vi "fgv_sessions.vi"(7 "Operation":T2(ring), 8 "error in":errorcluster, 10 "Session User Data in (None)":T1={"Instr type"="", "Instr type for err. msg."="", "Installed Options"=[], "OPC Timeout"=5000, "Query Instrument Status"=TRUE, "Check Range"=TRUE, "Check Options"=TRUE, "Add LF to Write"=TRUE, "Simulate"=FALSE, "Logging"=FALSE, "Logging params"=variant, "Interface Type"=enum."GPIB_VXI", "Fast Sweep"=0, "AdditionalFlags"=5000, "WaitBeforeWrite"=0, "WaitBeforeRead"=0, "BinDataChunkSize"=10000000} {"BinDataChunkSize" format="%.0p"; "AdditionalFlags" format="%08b"; "Fast Sweep" items=["Normal", "Fast"]}, 11 "VISA resource name":refnum<visa-resource-name>) -> (0 "error out":errorcluster, 2 "Session User Data out":T1={"Instr type"="", "Instr type for err. msg."="", "Installed Options"=[], "OPC Timeout"=5000, "Query Instrument Status"=TRUE, "Check Range"=TRUE, "Check Options"=TRUE, "Add LF to Write"=TRUE, "Simulate"=FALSE, "Logging"=FALSE, "Logging params"=variant, "Interface Type"=enum."GPIB_VXI", "Fast Sweep"=0, "AdditionalFlags"=5000, "WaitBeforeWrite"=0, "WaitBeforeRead"=0, "BinDataChunkSize"=10000000} {"BinDataChunkSize" format="%.0p"; "AdditionalFlags" format="%08b"; "Fast Sweep" items=["Normal", "Fast"]}, 3 "VISA resource name out":refnum<visa-resource-name> caption="VISA resource name")   [LabVIEW 2014, in "rszvl_rsidr_core.lvlib"]
uses:
  rszvl_rsidr_core.lvlib
  type_Session_Data.ctl
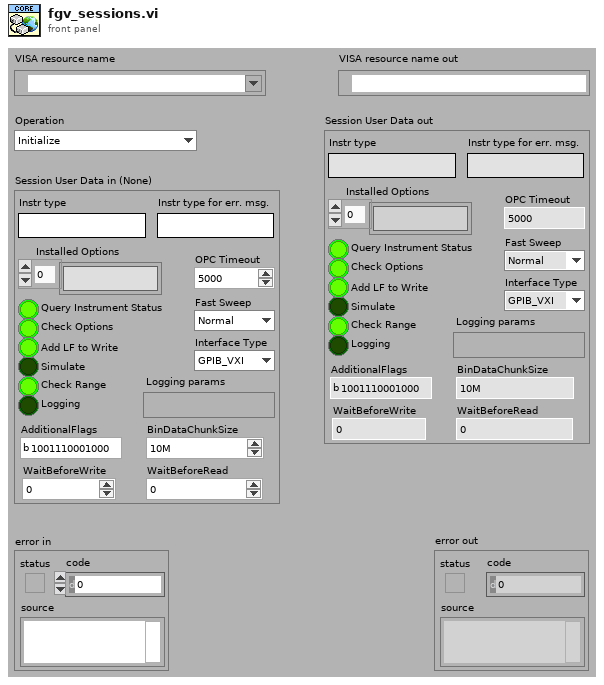
[diagram p1: front panel]
types:
  T1 = typedef "rszvl_rsidr_core.lvlib/type_Session_Data.ctl" = cluster{"Instr type":string, "Instr type for err. msg.":string, "Installed Options":string[], "OPC Timeout":i32, "Query Instrument Status":bool, "Check Range":bool, "Check Options":bool, "Add LF to Write":bool, "Simulate":bool, "Logging":bool, "Logging params":variant, "Interface Type":enum16{"Unknown", "GPIB", "VXI", "GPIB_VXI", "ASRL", "PXI", "TCPIP", "USB", "SOCKET"}, "Fast Sweep":i32, "AdditionalFlags":i32, "WaitBeforeWrite":i32, "WaitBeforeRead":i32, "BinDataChunkSize":i64}
  T2 = enum16{"Initialize", "GetData", "SetData", "Clear"}
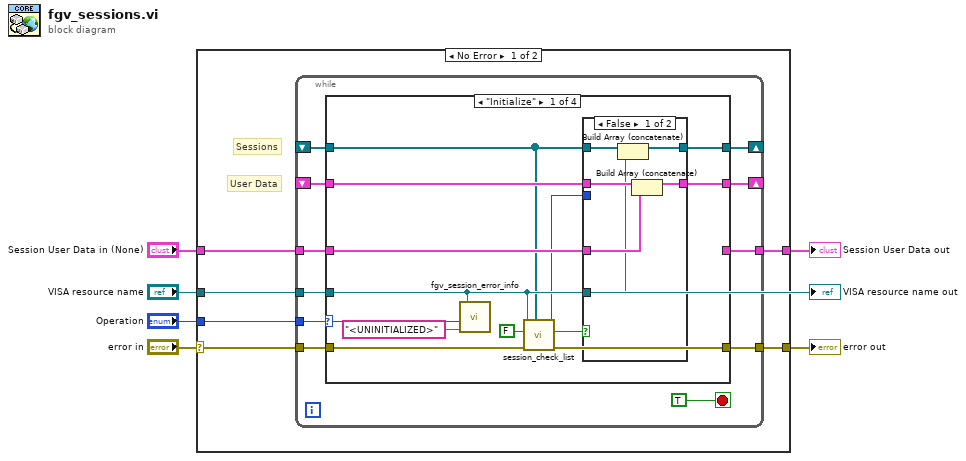
[diagram p0: block diagram]
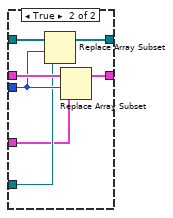
[diagram p2: hidden frame]
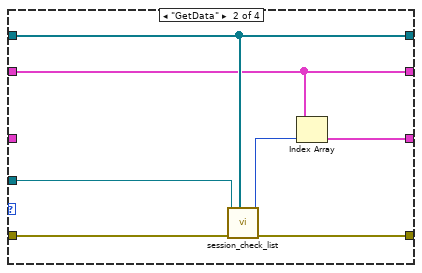
[diagram p3: hidden frame]
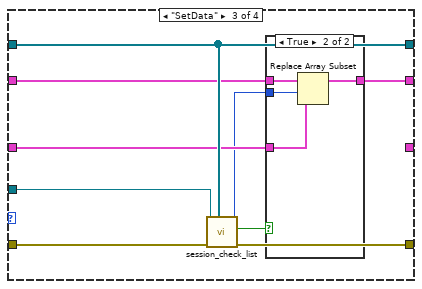
[diagram p4: hidden frame]
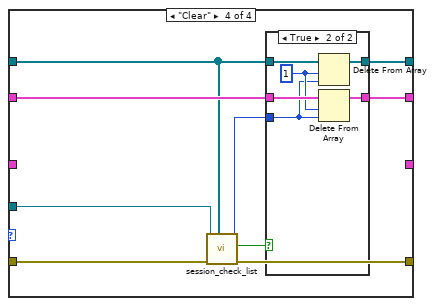
[diagram p6: hidden frame]
diagram:
  n1 = case shown="No Error" "error in" {
    selector: "error in" -> [w11 w88]
    tunnel: "Operation" -> [w8 _]
    tunnel: "Session User Data in (None)" -> [w9 _]
    tunnel: "VISA resource name" -> [w7 _]
    tunnel: [w12 _] -> w5
    tunnel: [w10 w88] -> w1
    frame No Error {
      # "User Data"
      # "Sessions"
      n2 = while {
        tunnel: [w13] -> w12
        tunnel: w11 -> [w16]
        tunnel: [w23] -> w10
        tunnel: w9 -> [w22]
        tunnel: w8 -> [w21]
        tunnel: w7 -> [w20]
        shift-right: [w18] -> _
        shift-left: _ -> [w19]
        shift-right: [w14] -> _
        shift-left: _ -> [w15]
        stop <- TRUE stop-if-true
        n3 = case "Operation case" shown="\"Initialize\"" w21 {
          selector: w21 -> [w25 _ _ _]
          tunnel: w20 -> [w26 w54 w64 w78]
          tunnel: w16 -> [w36 w56 w65 w79]
          tunnel: [w35 w55 w59 w77] -> w23
          tunnel: w19 -> [w30 w53 w63 w72]
          tunnel: w22 -> [w31 _ w61 _]
          tunnel: [w29 w53 w63 w71] -> w18
          tunnel: w15 -> [w32 w51 w62 w76]
          tunnel: [w28 w51 w60 w73] -> w14
          tunnel: [_ w52 _ _] -> w13
          frame "Initialize" {
            n4 = call "fgv_session_error_info.vi"("Session Error Info in (\"\")"="<UNINITIALIZED>" ("Session Error Info in (\"\")"), "Operation"=w25, "Session in"=w26) -> ()  [unwired: 4 in, 1 out]
            n5 = call "session_check_list.vi"("VISA resource names in"=w30, "error in"=w36, "Error if not found (T)"=FALSE, "VISA resource name"=w26) -> ("error out"=w35:errorcluster, "Found in the list"=w33:bool, "Session list index out"=w27:i32)  [unwired: 5 in]
            n6 = case shown="False" w33 {
              tunnel: w32 -> [w40 w49]
              tunnel: w31 -> [w39 w43]
              tunnel: w27 -> [_ w45]
              tunnel: w26 -> [w38 w44]
              tunnel: w30 -> [w42 w47]
              tunnel: [w41 w46] -> w29
              tunnel: [w37 w48] -> w28
              frame False {
                n7 = Build Array (concatenate)(w42, w38) -> (w41:refnum<visa-resource-name>[])
                n8 = Build Array (concatenate)(w40, w39) -> (w37:T1[])
              }
              frame True {
                n9 = Replace Array Subset(array=w47, new element=w44, index=w45) -> (w46:refnum<visa-resource-name>[])
                n10 = Replace Array Subset(array=w49, new element=w43, index=w45) -> (w48:T1[])
              }
            }
          }
          frame "GetData" {
            n11 = call "session_check_list.vi"("VISA resource names in"=w53, "error in"=w56, "VISA resource name"=w54) -> ("error out"=w55:errorcluster, "Session list index out"=w50:i32)  [unwired: 6 in, 1 out]
            n12 = Index Array(array=w51, index=w50) -> (element=w52:T1)
          }
          frame "SetData" {
            n13 = call "session_check_list.vi"("VISA resource names in"=w63, "error in"=w65, "VISA resource name"=w64) -> ("error out"=w59:errorcluster, "Found in the list"=w57:bool, "Session list index out"=w58:i32)  [unwired: 6 in]
            n14 = case shown="True" w57 {
              tunnel: w62 -> [w66 w70]
              tunnel: w61 -> [_ w67]
              tunnel: [w66 w69] -> w60
              tunnel: w58 -> [_ w68]
              frame False {
              }
              frame True {
                n15 = Replace Array Subset(array=w70, new element=w67, index=w68) -> (w69:T1[])
              }
            }
          }
          frame "Clear" {
            n16 = call "session_check_list.vi"("VISA resource names in"=w72, "error in"=w79, "VISA resource name"=w78) -> ("error out"=w77:errorcluster, "Found in the list"=w74:bool, "Session list index out"=w75:i32)  [unwired: 6 in]
            n17 = case shown="True" w74 {
              tunnel: w76 -> [w81 w85]
              tunnel: w75 -> [_ w82]
              tunnel: [w81 w84] -> w73
              tunnel: w72 -> [w80 w87]
              tunnel: [w80 w86] -> w71
              frame False {
              }
              frame True {
                w83 = 1 ("length")
                n18 = Delete From Array(array=w87, length=w83, index=w82) -> (array with subset deleted=w86:refnum<visa-resource-name>[])  [unwired: 1 out]
                n19 = Delete From Array(array=w85, length=w83, index=w82) -> (array with subset deleted=w84:T1[])  [unwired: 1 out]
              }
            }
          }
        }
      }
    }
    frame Error {
    }
  }
  "error out" <- w1
  "Session User Data out" <- w5
  "VISA resource name out" <- "VISA resource name"
